vi "FTW-Container-Object-Elements.vi"(0 "FTW-Container In":refnum<class "FTW-Container.lvclass">, 11 "error in":errorcluster) -> (4 "FTW-Container Out":refnum<class "FTW-Container.lvclass">, 6 "Names":string[](array[string]), 8 "Object Elements":refnum<class "FTW-Container.lvclass">[](array[class]), 15 "error out":errorcluster)   [LabVIEW 2018, in "FTW-Container.lvclass"]
uses:
  FTW-Container.lvclass
  FTW-Container.lvclass/FTW-Container.ctl
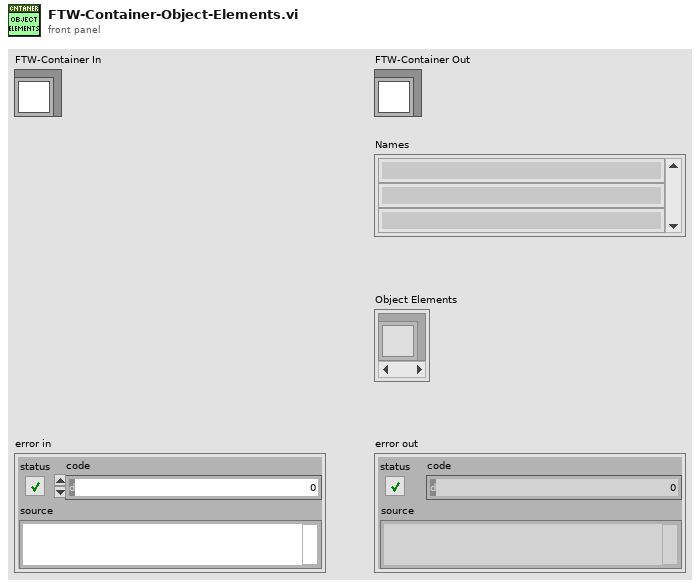
[diagram p1: front panel]
types:
  T1 = typedef "FTW-Container.lvclass/FTW-Container-Object.ctl" = cluster{"Names":string[], "Values":variant[]}
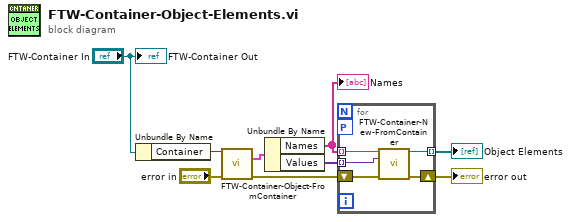
[diagram p0: block diagram]
diagram:
  n1 = Unbundle By Name("FTW-Container In") -> ("Container"=w4:variant)
  n2 = call "FTW-Container-Object-FromContainer.vi"("FTW-Container In"=w4, "error in"="error in") -> (6:w3:T1, "error out"=w6:errorcluster)  [unwired: 12 in]
  n3 = Unbundle By Name(w3) -> ("Names"=w2:string[], "Values"=w1:variant[])
  "Names" <- w2
  n4 = for {
    tunnel: [w12] -> w8 mode=indexing
    workers-P: _ -> [_]
    tunnel: w2 -> [w11] mode=indexing
    tunnel: w1 -> [w10] mode=indexing
    shift-right: [w13] -> w7
    shift-left: w6 -> [w14]
    n5 = call "FTW-Container-New-FromContainer.vi"("Name"=w11, "Container"=w10, "error in"=w14) -> ("FTW-Container"=w12:refnum<class "FTW-Container.lvclass">, "error out"=w13:errorcluster)  [unwired: 11 in]
  }
  "error out" <- w7
  "Object Elements" <- w8
  "FTW-Container Out" <- "FTW-Container In"
